vi "Update Case Result.vi"(8 "error in (no error)":errorcluster, 10 "Test Method Result":T1, 11 "Test Tree In":refnum<class "Test Result Tree V2.lvclass">) -> (0 "error out":errorcluster, 3 "Test Tree Out":refnum<class "Test Result Tree V2.lvclass">)   [LabVIEW 2020]
uses:
  Test Result Tree/Test Result Tree V2.lvclass
  C:/Git/astemes-lunit/source/Framework/Helper Classes/Test Tree/Test Tree.lvclass
  Framework/Result Types/Case Result/Test Case Result.ctl
  Framework/Result Types/Method Result/Method Result.ctl
  Result/Status.ctl
  Framework/Result Types/Assertion Result/Assertion Result.ctl
  Framework/Result Types/Assertion Result/Public/TypeDefs/Assertion Type.ctl
  Framework/Helper Classes/Test Tree/Test Tree.lvclass/Test Tree.ctl
  Framework/Result Types/Case Result/Private/Merge Status.vi
  Test Result Tree/Test Result Tree V2.lvclass/Test Result Tree V2.ctl
  Framework/Result Types/Case Result/Test Case Result.lvlib
  Framework/Helper Classes/Test Tree/Test Tree.lvclass
  Framework/Result Types/Assertion Result/Assertion Result.lvlib
  Framework/Result Types/Method Result/Method Result.lvlib
  Result/Result.lvlib
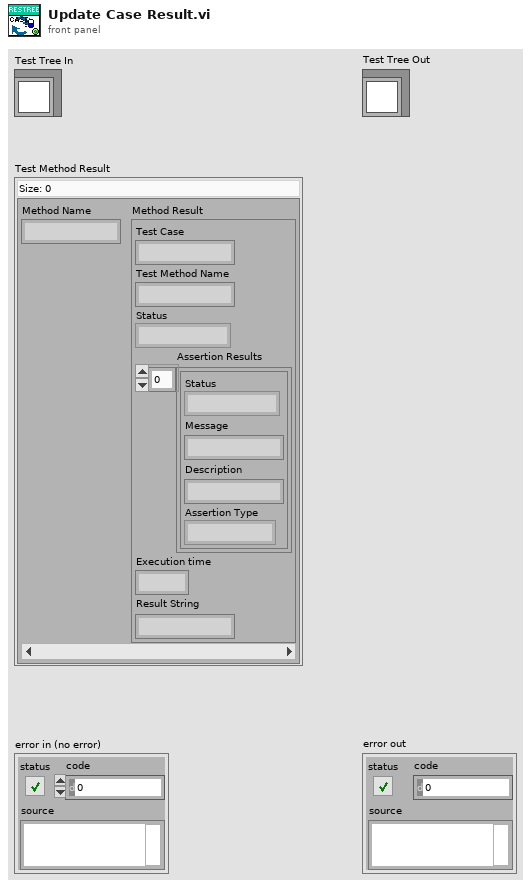
[diagram p1: front panel]
types:
  T1 = typedef "Test Case Result.lvlib/Test Case Result.ctl" = map{string, T2}
  T2 = typedef "Method Result.lvlib/Method Result.ctl" = cluster{"Test Case":string, "Test Method Name":string, "Status":T3, "Assertion Results":T4[], "Execution time":dbl, "Result String":string}
  T3 = typedef "Result.lvlib/Status.ctl" = enum16{"Passed", "Failed", "Error", "Skipped", "Setup Error", "Broken", "Teardown Error"}
  T4 = typedef "Assertion Result.lvlib/Assertion Result.ctl" = cluster{"Status":T3, "Message":string, "Description":string, "Assertion Type":T5}
  T5 = typedef "Result.lvlib/Assertion Type.ctl" = enum16{"None", "Pass", "Fail", "Skip", "Pass if Equal", "Fail if Equal", "Pass if Error", "Fail if Error", "Pass if", "Fail if"}
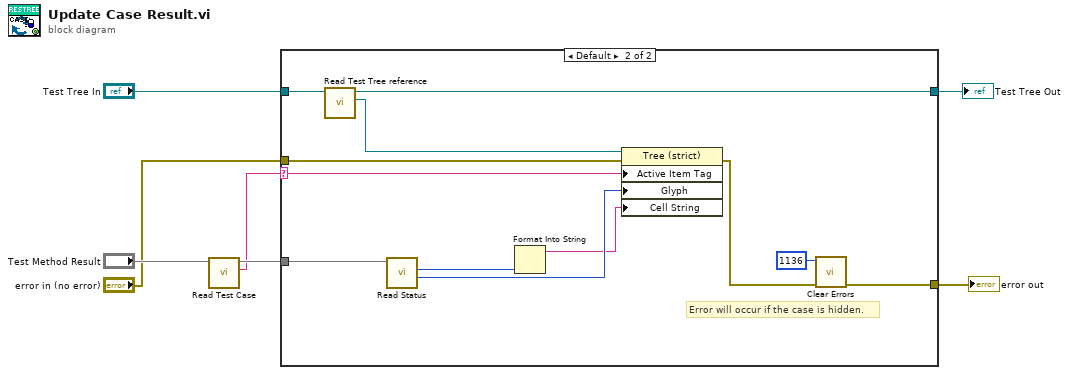
[diagram p0: block diagram]
diagram:
  n1 = call "Read Test Case.vi"("Test Case Result In"="Test Method Result") -> ("Test Case"=w2:string, "Test Case Result Out"=w4:T1)  [unwired: 9 in]
  n2 = case shown="Default" w2 {
    selector: w2 -> [_ w16]
    tunnel: "Test Tree In" -> [w9 w12]
    tunnel: [w9 w13] -> w5
    tunnel: w4 -> [_ w19]
    tunnel: [w8 w15] -> w3
    tunnel: "error in (no error)" -> [w8 w10]
    frame "" {
    }
    frame Default {
      # "Error will occur if the case is hidden."
      n3 = call "Read Test Tree reference.vi"("Test Tree in"=w12) -> ("Test Tree reference"=w11:refnum<vi>, "Test Tree out"=w13:refnum<class "Test Result Tree V2.lvclass">)  [unwired: 8 in, 1 out]
      n4 = call "Read Status.vi"("Test Case Result In"=w19) -> ("Glyph Index"=w20:i32, "Status"=w21:T3)  [unwired: 8 in, 1 out]
      n5 = Format Into String(w21) -> (resulting string=w18:string)  [unwired: 3 in, 1 out]
      n6 = property class="Tree (strict)"(reference=w11, error in=w10, "Active Item Tag"=w16, "Glyph"=w20, "Cell String"=w18) -> (error out=w17:errorcluster)  [unwired: 1 out]
      n7 = call <vilib>:"Clear Errors.vi"("error in (no error)"=w17, "specific error code to clear (0: all)"=1136) -> ("error out"=w15:errorcluster)  [unwired: 4 in, 1 out]
    }
  }
  "error out" <- w3
  "Test Tree Out" <- w5
